vi "ttm_stopLogging_poller.vi"() -> ()   [LabVIEW 2009]
panel:
  in  "Interval/Buffer Parameters":T1={"Sample interval - ms (2)"=2.0, "Buffer Length (1000)"=1000, "No. of Buffers (0)"=0} {"Sample interval - ms (2)" min=0.2 format="%.1f"}
  # "datalogger internal \npreferences:"
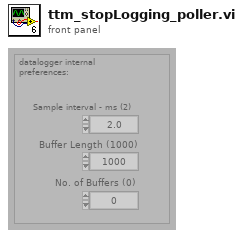
[diagram p1: front panel]
types:
  T1 = cluster{"Sample interval - ms (2)":dbl, "Buffer Length (1000)":i32, "No. of Buffers (0)":i32}
  T2 = cluster{"Device ID":i32, "Device Name":string, "Device Type":i32}[]
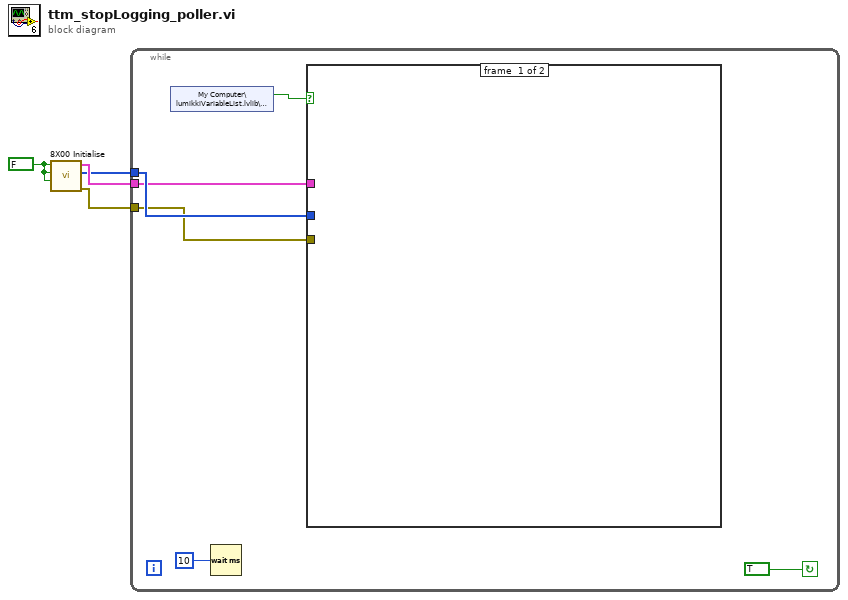
[diagram p0: block diagram]
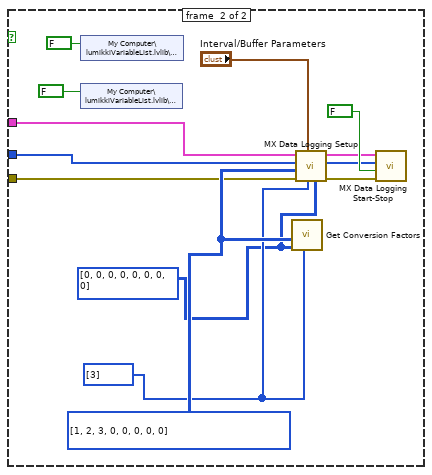
[diagram p2: hidden frame]
diagram:
  w4 = FALSE ("Create Console? (T)")
  n1 = call "8X00 Initialise.vi"("Reset?"=w4, "Create DVM? (T)"=w4, "Create Console? (T)"=w4) -> ("error out"=w1:errorcluster, "Axis Selector"=w2:i32[], "Axis Information"=w3:T2)  [unwired: 1 in, 1 out]
  n2 = while {
    tunnel: w3 -> [w9]
    tunnel: w2 -> [w10]
    tunnel: w1 -> [w8]
    stop <- TRUE continue-if-true
    n3 = shared-variable "My Computer\\lumikkiVariableList.lvlib\\stopLogging"() -> (w5:bool)  [unwired: 1 in, 1 out]
    n4 = Wait (ms)(milliseconds to wait=u32 10) -> ()  [unwired: 1 out]
    n5 = case shown="True" w5 {
      tunnel: w10 -> [_ w15]
      tunnel: w9 -> [_ w14]
      tunnel: w8 -> [_ w13]
      frame #0 {
      }
      frame #1 {
        w22 = i32[] [3] ("Number of Columns")
        w21 = i32[][] [[0, 0, 0, 0, 0, 0, 0, 0]] items=["Feedback", "Direct Auxilary"] ("Column Types")
        w23 = i32[][] [[1, 2, 3, 0, 0, 0, 0, 0]] items=["Not Used", "Channel 1/Logging time", "Channel 2/Controlling command", "Channel 3/Controlling error", "Channel 4/Elapsed quarter-cycle counter", "Total accumulated quarter-cycle counter", "Elapsed segment counter", "Total accumulated segment counter", "Servovalve drive", "Block count", "Uncompensated servovalve drive", "Geometric compensation output 1", "Geometric compensation output 2", "Re-Sampling Filter 1", "Re-Sampling Filter 2", "Re-Sampling Filter 3", "Re-Sampling Filter 4", "Outer cascaded controller output", "Delta_P or acceleration compensation (Raw)", "Auxiliary input from the front of the IAC", "Waveform identifier", "Reserved", "Digital I/O and sample playback actions", "Reserved", "Motor current (EIB only)", "Motor instantaneous power (EIB only)", "Motot filtered power (EIB only)", "Motor speed (EIB only)", "Motor viscous loss (EIB only)"] ("Column Channels")
        n6 = shared-variable "My Computer\\lumikkiVariableList.lvlib\\stopLogging"(FALSE ("stopLogging")) -> ()  [unwired: 1 in, 1 out]
        n7 = shared-variable "My Computer\\lumikkiVariableList.lvlib\\loggingIsOn"(FALSE ("stopLogging")) -> ()  [unwired: 1 in, 1 out]
        n8 = call "Get Conversion Factors.vi"("Column Channels"=w23, "Column Types"=w21, "Number of Columns"=w22) -> ()  [unwired: 2 in, 1 out]
        n9 = call "MX Data Logging Setup.vi"("Column Types"=w21, "Number of Columns"=w22, "Interval/Buffer Parameters"="Interval/Buffer Parameters", "error in (no error)"=w13, "Column Channels"=w23, "Axis Selector"=w15, "Axis Information"=w14) -> ("error out"=w16:errorcluster, "Axis Selector copy"=w17:i32[], "Axis Information out"=w18:T2)  [unwired: 1 out]
        n10 = call "MX Data Logging Start-Stop.vi"("error in (no error)"=w16, "Start (T)"=FALSE, "Axis Selector"=w17, "Axis Information"=w18) -> ()  [unwired: 4 in, 3 out]
      }
    }
  }
